vi "DeInit.vi"(8 "error in (no error)":errorcluster, 11 "DongWoo in":refnum<class "DongWoo.lvclass">) -> (0 "error out":errorcluster, 3 "DongWoo out":refnum<class "DongWoo.lvclass">)   [LabVIEW 2023, in "DongWoo_Spectrometer.lvlib" / "DongWoo.lvclass"]
uses:
  DongWoo.lvclass
  DongWoo.lvclass/DongWoo.ctl
  <vilib>/Instr/_visa.llb/Select Event Type.ctl
  <vilib>/ActorFramework/Stop Msg/Stop Msg.lvclass
  <vilib>/ActorFramework/Actor/Actor.lvclass
  C:/Program Files/National Instruments/LabVIEW 2023/vi.lib/ActorFramework/Actor/Actor.lvclass
  C:/Users/DELL/Documents/LVDAQ/ConcreteClasses/ConcreteInstrumentClasses/SpectrometerClasses/DongWoo_LV/DongWoo/DongWoo.lvclass
  C:/Users/DELL/Documents/LVDAQ/Interfaces/InitDeinitInterface/InitDeinit/InitDeinit.lvclass
  C:/Users/DELL/Documents/LVDAQ/Interfaces/AbstractInstrumentClasses/Spectrometers_LV/SpectrometerInterface/Spectrometer.lvclass
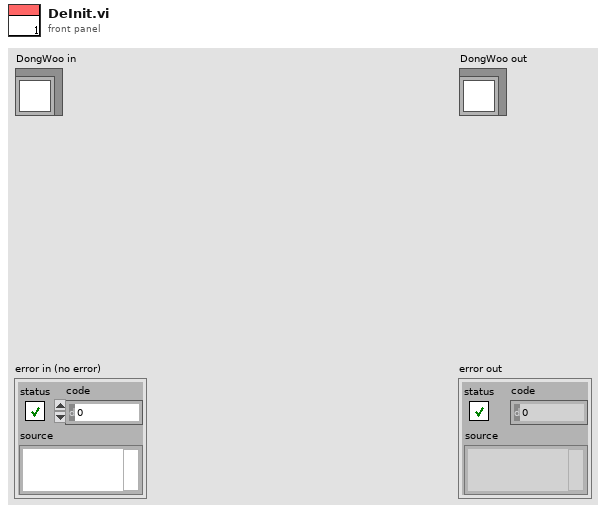
[diagram p1: front panel]
types:
  T1 = typedef "Select Event Type.ctl" = u32
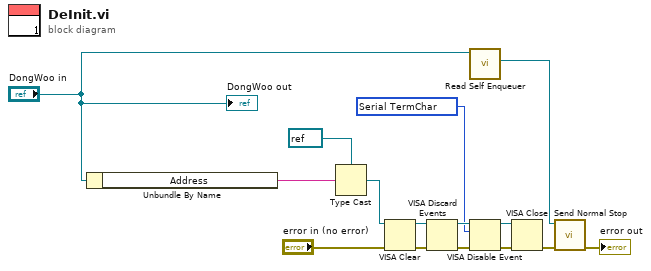
[diagram p0: block diagram]
diagram:
  w9 = T1 1073684516 items=["Service Request"=1073684491, "Trigger"=3221168138, "Clear"=1073684493, "VXI Signal"=1073684512, "VXI/VME Interrupt"=3221168161, "VXI/VME Sysfail"=1073684509, "VXI/VME Sysreset"=1073684510, "GPIB CIC"=1073684498, "GPIB Talk"=1073684499, "GPIB Listen"=1073684500, "PXI Interrupt"=1073684514, "Serial Break"=1073684515, "Serial TermChar"=1073684516, "Serial CTS"=1073684521, "Serial DSR"=1073684522, "Serial DCD"=1073684524, "Serial RI"=1073684526, "Serial Character"=1073684533, "USB Interrupt"=1073684535, "All Enabled"=1073709055] ("Event Type")
  n1 = Unbundle By Name("DongWoo in") -> ("Address"=w7:string)
  n2 = Type Cast(type=refnum<visa-resource-name> refnum ("VISA resource name"), x=w7) -> (*(type *) &x=w6:refnum<visa-resource-name>)
  n3 = VISA Clear(VISA resource name=w6, error in (no error)="error in (no error)") -> (VISA resource name out=w13:refnum<visa-resource-name>, error out=w11:errorcluster)
  n4 = VISA Discard Events(8:w11, 11:w13) -> (0:w14:errorcluster, 3:w15:refnum<visa-resource-name>)  [unwired: 2 in]
  n5 = call <vilib>:"Read Self Enqueuer.vi"("Actor"="DongWoo in") -> ("Self Enqueuer"=w4:refnum<class "Message Enqueuer.lvclass">)  [unwired: 10 in]
  n6 = VISA Disable Event(8:w14, 10:w9, 11:w15) -> (0:w10:errorcluster, 3:w12:refnum<visa-resource-name>)  [unwired: 1 in]
  n7 = VISA Close(VISA resource name=w12, error in (no error)=w10) -> (error out=w5:errorcluster)
  n8 = call <vilib>:"Send Normal Stop.vi"("error in (no error)"=w5, "Message Enqueuer"=w4) -> ("error out"=→"error out":errorcluster)  [unwired: 9 in]
  "DongWoo out" <- "DongWoo in"
